vi "Engine Out - GDI - Faults.vi"(11 "Control Inputs":T1={"Engine Speed [RPM]"=0.0, "Engine Status"=enum."STALLED", "Load Control \nMode"=enum."High-Idle Governor", "dt(s)"=0.0, "Number of Cylinders"=0, "Engine Displacement [cc]"=0.0, "StoichAFR"=0.0, "Q.LHV Fuel [kJ/kg]"=0.0, "BattV PSU [V]"=0.0, "12V PSU [V]"=0.0, "5V PSU [V]"=0.0, "Pedal Position [%]"=0.0, "Oil Pressure [kPa]"=0.0, "Oil Temp [C]"=0.0, "Oil Level [%]"=0.0, "Engine Coolant Temp (ECT) [C]"=0.0, "Engine Coolant Pressure [kPa]"=0.0, "Rail Pressure [bar]"=0.0, "Fuel Pressure [kPa]"=0.0, "Fuel Temp [C]"=0.0, "Vacuum Pressure [kPa]"=0.0, "Throttle Position [%]"=0.0, "Cam1 Advance [CAD]"=0.0, "Cam2 Advance [CAD]"=0.0, "Cam3 Advance [CAD]"=0.0, "Cam4 Advance [CAD]"=0.0, "CA50 Control Output [CAD]"=[], "CA50 Control Output Valid"=[], "Intake Air Temp (IAT) [C]"=0.0, "Barometric Air Pressure [kPa]"=0.0, "Intake Air Rel. Humidity [%]"=0.0, "Mass Air Flow (MAF) [kg/hr]"=0.0, "Turbo Inlet Air Pressure [kPa]"=0.0, "Turbo Inlet Air Temp [C]"=0.0, "Turbo Outlet Air Pressure [kPa]"=0.0, "Turbo Outlet Air Temp [C]"=0.0, "CAC Outlet Pressure [kPa]"=0.0, "CAC Outlet Temp [C]"=0.0, "Intake Manifold Pressure (MAP) [kPa]"=0.0, "Intake Manifold Temp (MAT) [C]"=0.0, "Exhaust Manifold Pressure [kPa]"=0.0, "Exhaust Manifold Temp [C]"=0.0, "HighP EGR Cooler Outlet Pressure [kPa]"=0.0, "HighP EGR Cooler Outlet Temp [C]"=0.0, "HighP EGR Differential Pressure [kPa]"=0.0, "HighP EGR Valve Position [%]"=0.0, "Turbo Outlet Exhaust Pressure [kPa]"=0.0, "Turbo Outlet Exhaust Temp [C]"=0.0, "VGT Position 1 [%]"=0.0, "VGT Position 2 [%]"=0.0, "Turbo Speed 1 [RPM]"=0.0, "Turbo Speed 2 [RPM]"=0.0, "LowP EGR Differential Pressure [kPa]"=0.0, "LowP EGR Valve Position [%]"=0.0, "UEGO1Lambda"=0.0, "UEGO1_Hot"=FALSE, "UEGO2Lambda"=0.0, "UEGO2_Hot"=FALSE, "Knock Intensity"=[], "Knock"=[]} {"Knock Intensity" format="%.2f"; "CA50 Control Output [CAD]" format="%.2f"; "Exhaust Manifold Temp [C]" format="%#_6f"; "UEGO2Lambda" format="%.2f"; "Intake Manifold Temp (MAT) [C]" format="%#_6f"; "UEGO1Lambda" format="%.2f"}) -> ()   [LabVIEW 2015, in "ECS-RT.lvlib"]
uses:
  ECS-RT.lvlib
  Typedefs/Control Inputs/Control Inputs.ctl
  Typedefs/EPT/Engine Status.ctl
  Typedefs/MISC/Load Control Mode.ctl
  ECS-Shared.lvlib
types:
  T1 = typedef "ECS-Shared.lvlib/Control Inputs.ctl" = cluster{"Engine Speed [RPM]":sgl, "Engine Status":T2, "Load Control \nMode":T3, "dt(s)":sgl, "Number of Cylinders":u8, "Engine Displacement [cc]":sgl, "StoichAFR":sgl, "Q.LHV Fuel [kJ/kg]":sgl, "BattV PSU [V]":sgl, "12V PSU [V]":sgl, "5V PSU [V]":sgl, "Pedal Position [%]":sgl, "Oil Pressure [kPa]":sgl, "Oil Temp [C]":sgl, "Oil Level [%]":sgl, "Engine Coolant Temp (ECT) [C]":sgl, "Engine Coolant Pressure [kPa]":sgl, "Rail Pressure [bar]":sgl, "Fuel Pressure [kPa]":sgl, "Fuel Temp [C]":sgl, "Vacuum Pressure [kPa]":sgl, "Throttle Position [%]":sgl, "Cam1 Advance [CAD]":sgl, "Cam2 Advance [CAD]":sgl, "Cam3 Advance [CAD]":sgl, "Cam4 Advance [CAD]":sgl, "CA50 Control Output [CAD]":sgl[], "CA50 Control Output Valid":bool[], "Intake Air Temp (IAT) [C]":sgl, "Barometric Air Pressure [kPa]":sgl, "Intake Air Rel. Humidity [%]":sgl, "Mass Air Flow (MAF) [kg/hr]":sgl, "Turbo Inlet Air Pressure [kPa]":sgl, "Turbo Inlet Air Temp [C]":sgl, "Turbo Outlet Air Pressure [kPa]":sgl, "Turbo Outlet Air Temp [C]":sgl, "CAC Outlet Pressure [kPa]":sgl, "CAC Outlet Temp [C]":sgl, "Intake Manifold Pressure (MAP) [kPa]":sgl, "Intake Manifold Temp (MAT) [C]":sgl, "Exhaust Manifold Pressure [kPa]":sgl, "Exhaust Manifold Temp [C]":sgl, "HighP EGR Cooler Outlet Pressure [kPa]":sgl, "HighP EGR Cooler Outlet Temp [C]":sgl, "HighP EGR Differential Pressure [kPa]":sgl, "HighP EGR Valve Position [%]":sgl, "Turbo Outlet Exhaust Pressure [kPa]":sgl, "Turbo Outlet Exhaust Temp [C]":sgl, "VGT Position 1 [%]":sgl, "VGT Position 2 [%]":sgl, "Turbo Speed 1 [RPM]":sgl, "Turbo Speed 2 [RPM]":sgl, "LowP EGR Differential Pressure [kPa]":sgl, "LowP EGR Valve Position [%]":sgl, "UEGO1Lambda":sgl, "UEGO1_Hot":bool, "UEGO2Lambda":sgl, "UEGO2_Hot":bool, "Knock Intensity":sgl[], "Knock":bool[]}
  T2 = typedef "ECS-Shared.lvlib/Engine Status.ctl" = enum16{"OFF", "STALLED", "CRANKING", "RUNNING", "ACCEL", "DECEL", "SAFE"}
  T3 = typedef "ECS-Shared.lvlib/Load Control Mode.ctl" = enum16{"No Governor", "Low-Idle Governor", "High-Idle Governor"}
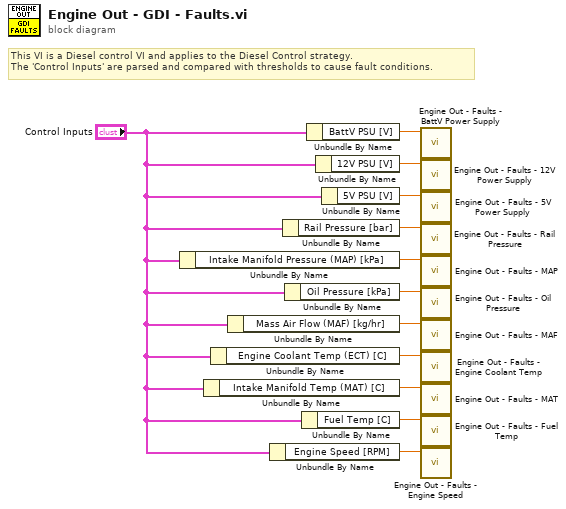
[diagram p0: block diagram]
diagram:
  # "This VI is a Diesel control VI and applies to the Diesel Control strategy.  \nThe 'Control Inputs' are parsed and compared with thresholds to cause fault conditions."
  n1 = Unbundle By Name("Control Inputs") -> ("Intake Manifold Pressure (MAP) [kPa]"=w5:sgl)
  n2 = Unbundle By Name("Control Inputs") -> ("Intake Manifold Temp (MAT) [C]"=w2:sgl)
  n3 = Unbundle By Name("Control Inputs") -> ("Engine Coolant Temp (ECT) [C]"=w8:sgl)
  n4 = Unbundle By Name("Control Inputs") -> ("Mass Air Flow (MAF) [kg/hr]"=w7:sgl)
  n5 = Unbundle By Name("Control Inputs") -> ("Engine Speed [RPM]"=w10:sgl)
  n6 = Unbundle By Name("Control Inputs") -> ("Rail Pressure [bar]"=w4:sgl)
  n7 = Unbundle By Name("Control Inputs") -> ("Oil Pressure [kPa]"=w6:sgl)
  n8 = Unbundle By Name("Control Inputs") -> ("Fuel Temp [C]"=w9:sgl)
  n9 = Unbundle By Name("Control Inputs") -> ("BattV PSU [V]"=w12:sgl)
  n10 = Unbundle By Name("Control Inputs") -> ("12V PSU [V]"=w11:sgl)
  n11 = Unbundle By Name("Control Inputs") -> ("5V PSU [V]"=w3:sgl)
  n12 = call "Engine Out - Faults - BattV Power Supply.vi"("BattV [V]"=w12) -> ()  [unwired: 11 in]
  n13 = call "Engine Out - Faults - 12V Power Supply.vi"("12V PSU [V]"=w11) -> ()  [unwired: 11 in]
  n14 = call "Engine Out - Faults - 5V Power Supply.vi"("5V PSU [V]"=w3) -> ()  [unwired: 11 in]
  n15 = call "Engine Out - Faults - Rail Pressure.vi"("RailP [bar]"=w4) -> ()  [unwired: 11 in]
  n16 = call "Engine Out - Faults - MAP.vi"("Intake Manifold Pressure [kPa]"=w5) -> ()  [unwired: 11 in]
  n17 = call "Engine Out - Faults - Oil Pressure.vi"("OilP [kPa]"=w6) -> ()  [unwired: 11 in]
  n18 = call "Engine Out - Faults - MAF.vi"("MAF [kg/hr]"=w7) -> ()  [unwired: 11 in]
  n19 = call "Engine Out - Faults - Engine Coolant Temp.vi"("Engine Coolant Temp [C]"=w8) -> ()  [unwired: 11 in]
  n20 = call "Engine Out - Faults - MAT.vi"("Intake Manifold Temperature [C]"=w2) -> ()  [unwired: 11 in]
  n21 = call "Engine Out - Faults - Fuel Temp.vi"("Fuel Temp [C]"=w9) -> ()  [unwired: 11 in]
  n22 = call "Engine Out - Faults - Engine Speed.vi"("Engine Speed [RPM]"=w10) -> ()  [unwired: 11 in]
